vi "Destroy.vi"(0 "reference":refnum<class "UseCaseNode.lvclass">, 5 "error in (no error)":errorcluster) -> (14 "reference out":refnum<class "UseCaseNode.lvclass">, 19 "error out":errorcluster)   [LabVIEW 2014, in "UseCaseNode.lvclass"]
doc: "Destroys a UseCaseNode object created with a UseCaseNode constructor VI.\n\n[GOOP 2.1]"
uses:
  <resource>/Framework/Providers/Open_GDS/UML/UseCaseNode_class/UseCaseNode.lvclass
  <resource>/Framework/Providers/Open_GDS/UML/RectangularNode_class/RectangularNode.lvclass
  <resource>/Framework/Providers/Open_GDS/UML/MultiLineString_class/MultiLineString.lvclass
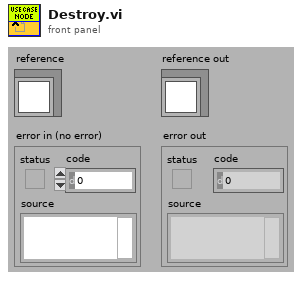
[diagram p1: front panel]
types:
  T1 = typedef "UseCaseNode.lvclass/ObjectAttributes.ctl" = cluster{"name":refnum<class "MultiLineString.lvclass">, "DEFAULT_WIDTH":i32, "DEFAULT_HEIGHT":i32}
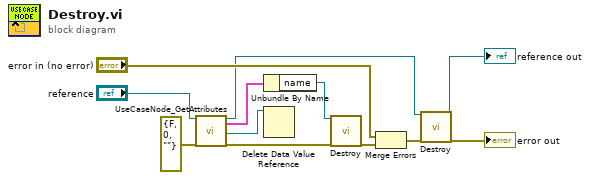
[diagram p0: block diagram]
diagram:
  n1 = call <resource>:"UseCaseNode_GetAttributes.vi"("reference in"="reference", "error in (no error)"=errorcluster {"status"=FALSE, "code"=0, "source"=""}) -> ("reference out"=w2:refnum<class "UseCaseNode.lvclass">, "Data"=w4:T1, "DataRef"=w3:refnum<data-value>, "error out"=w6:errorcluster)  [unwired: 1 in, 13 out]
  n2 = Unbundle By Name(w4) -> ("name"=w8:refnum<class "MultiLineString.lvclass">)
  n3 = Delete Data Value Reference(data value reference=w3) -> ()  [unwired: 1 in, 2 out]
  n4 = call-dynamic "Destroy.vi"("reference"=w8, "error in (no error)"=w6) -> ("error out"=w7:errorcluster)  [unwired: 16 in, 1 out]
  n5 = Merge Errors("error in (no error)", w7) -> (w5:errorcluster)
  n6 = call-parent "Destroy.vi"("reference"=w2, "error in (no error)"=w5) -> ("reference out"=→"reference out":refnum<class "UseCaseNode.lvclass">, "error out"=→"error out":errorcluster)  [unwired: 16 in]
